vi "选择开关（波段开关）.vi"() -> ()   [LabVIEW 2012]
panel:
  out "量表":u8(knob) scale=0.0..3.0
  in  "旋钮":u8(knob) scale=0.0..3.0
  in  "风扇速度波段开关":u8(slide) scale=0.0..3.0
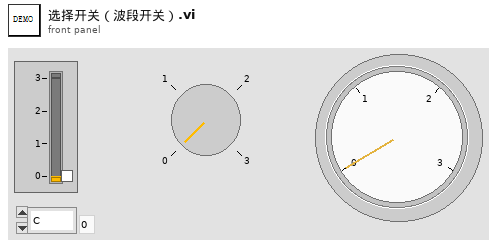
[diagram p1: front panel]
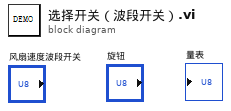
[diagram p0: block diagram]
diagram:
